vi "PS35_JoyZeroX.vi"(0 "Control unit ID":i32=1 min=1 max=10, 1 "function":bool, 2 "Value-In":i32=512 min=0 max=1023, 3 "error in (no error)":errorcluster) -> (7 "Value-Out":i32, 9 "error out":errorcluster)   [LabVIEW 2020]
doc: "PS35_JoyZeroX.vi, created: 05.03.2009 alex; last change: 22.10.2019 alex;\n\n<B>FUNCTIONS:</B> \n\n<B>Read:</B> FALSE: read zero point of the joystick plane X.\n<B>Write:</B> TRUE: set zero point of the joystick plane X.\n----------------------------------------------------------------------------------------\n<B>INPUT:</B>\n[TF] <B>function:</B> function selector. (Read, Write)\n[I32] <B>Control unit ID:</B> control unit index. (Default=1, Range=1...10) \n[I32] <B>Value-In:</B> zero point. (only for Write: Default=512, Range=0...1023)\n[CLU] <B>error in</B>\n----------------------------------------------------------------------------------------\n<B>OUTPUT:</B>\n[I32] <B>Value-Out:</B> zero point. (for Write: Value-Out=Value-In) \n[CLU] <B>error out</B>\n----------------------------------------------------------------------------------------\n<B>SUB-VIs:</B>\nPS35_GetReadError.vi\n----------------------------------------------------------------------------------------\n<B>EXT-Calls:</B>\nps35.dll (V2.01)\n----------------------------------------------------------------------------------------"
uses:
  ps35.dll
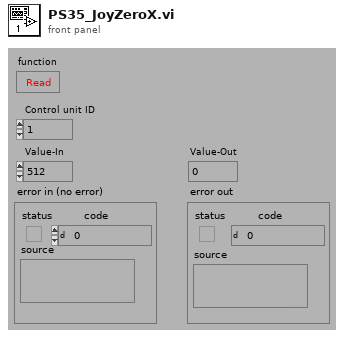
[diagram p1: front panel]
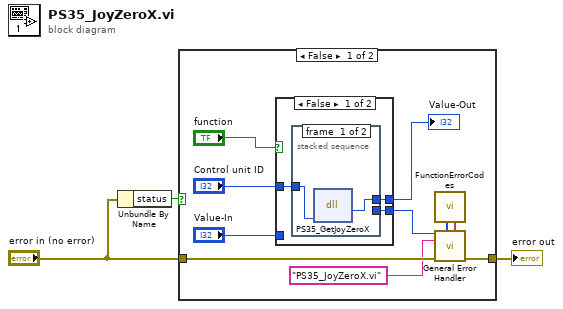
[diagram p0: block diagram]
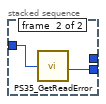
[diagram p2: hidden frame]
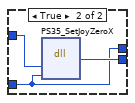
[diagram p3: hidden frame]
diagram:
  n1 = Unbundle By Name("error in (no error)") -> ("status"=w1:bool)
  n2 = case shown="False" w1 {
    tunnel: "error in (no error)" -> [w13 w24]
    tunnel: [w12 w24] -> w3
    frame False {
      n3 = case shown="False" "function" {
        tunnel: "Control unit ID" -> [w15 w22]
        tunnel: [w16 w23] -> w9
        tunnel: "Value-In" -> [_ w21]
        tunnel: [w14 w21] -> w7
        frame False {
          n4 = stacked-sequence {
            tunnel: [_ w20] -> w16
            tunnel: w15 -> [w18 w19]
            tunnel: [w17 _] -> w14
            frame #0 {
              n5 = dll-call lib="C:/GEECS/Developers Version/source/Device Drivers/OwiSoft/OWISoftOEM/ps35/labview/lv82/ps35.dll" fn="PS35_GetJoyZeroX" label="PS35_Get\nJoyZeroX"("Index"=w18) -> ("Rückgabetyp"=w17:i32)  [unwired: 4 in, 2 out]
            }
            frame #1 {
              n6 = call "PS35_GetReadError.vi"("Control unit ID"=w19) -> ("Read error"=w20:i32)
            }
          }
        }
        frame True {
          n7 = dll-call lib="C:/GEECS/Developers Version/source/Device Drivers/OwiSoft/OWISoftOEM/ps35/labview/lv82/ps35.dll" fn="PS35_SetJoyZeroX" label="PS35_Set\nJoyZeroX"("Index"=w22, "Value"=w21) -> ("Rückgabetyp"=w23:i32)  [unwired: 5 in, 2 out]
        }
      }
      "Value-Out" <- w7
      n8 = call "FunctionErrorCodes.vi"() -> ("[user-defined codes]"=w5:i32[], "[user-defined descriptions]"=w4:string[])  [unwired: 8 in]
      n9 = call <vilib>:"General Error Handler.vi"("[error code] (0)"=w9, "[user-defined codes]"=w5, "[user-defined descriptions]"=w4, "[error source] (\" \")"="PS35_JoyZeroX.vi" ("[error source] (\" \")"), "error in (no error)"=w13) -> ("error out"=w12:errorcluster)  [unwired: 6 in, 4 out]
    }
    frame True {
    }
  }
  "error out" <- w3
